vi "paper1.vi"() -> ()   [LabVIEW 2019]
uses:
  <vilib>/BLE/type_def/address_type.ctl
panel:
  out "check time elapsed (S)":dbl
  in  "Tab Control":T1(tab)
  in  "both 3":path=path "C:/Users/Admin/Desktop/Asfand/Working Examples dont edit/7_audio random indicator/both.wav"
  in  "left 2":path=path "C:/Users/Admin/Desktop/Asfand/Working Examples dont edit/7_audio random indicator/left.wav"
  in  "right 3":path=path "C:/Users/Admin/Desktop/Asfand/Working Examples dont edit/7_audio random indicator/right.wav"
  out "BLED112 Dongle Info":string
  in  "COM Bluegiga in":refnum<visa-resource-name>="COM3"
  in  "Address Type":T2=1 items=["Public", "Random"]
  in  "MAC Address":string="F7:AE:10:9A:D9:38"
  out "Scanning":bool
  out "Connected":bool
  out "User input history":string[](array[string])
  out "right 4":i16[](array[numeric])
  out "left 3":i16[](array[numeric])
  out "both":i16[](array[numeric])
  out "Seconds that the game lasted.":dbl
  out "total commands":i32
  out "timer started?":bool
  in  "savefile":path=path "C:/Users/Admin/Desktop/experiment results/name_test1.xlsx" caption="Filename"
  out "possible decisions":string[](array[string])
  out "result":i16
  out "uuid loop":i32
  out "stimulii section precursor":bool
  out "LARGE LOOP":i32
  out "INSIDE RANDOM LOOP":i16
  out "Post trigger response?":bool
  out "Trigger checked?":bool
  out "UUID START":bool
  out "Stimulii section":bool
  out "Stimulii Given?":bool
  out "Number of moves loop":i32
  in  "Right threshold real time update":dbl(slide)=40.2088948787062 scale=0.0..255.0
  out "right":u8(graph)
  out "left":u8(graph)
  out "Left Eye element (PIN A0)":u8
  out "Right Eye Element (PIN A1)":u8
  out "DECISION LOOP":i32
  out "last eye movement":string
  out "Post-Trigger Detection":string
  in  "left threshod real time update":dbl(slide)=40.58355437665783 scale=0.0..255.0
  out "Game finished?":bool=TRUE
  out "Trigger  right eye":bool
  out "right-":bool
  out "Left-":bool
  out "both-":bool
  out "Both":bool
  out "Left":bool
  out "Right":bool
  # "1.Blink both eyes to initiate trigger,\n then blink as stimulii.\n2. If the led user input led does not turn on. \n(try blinking again, a faster response can do the trick)\n3. There will be 20 commands. \n4. moving your head will triger a response.  (slow and small movment will not)\n5. When 20 commands are registered (with triggers) then game finished \nwill turn red"
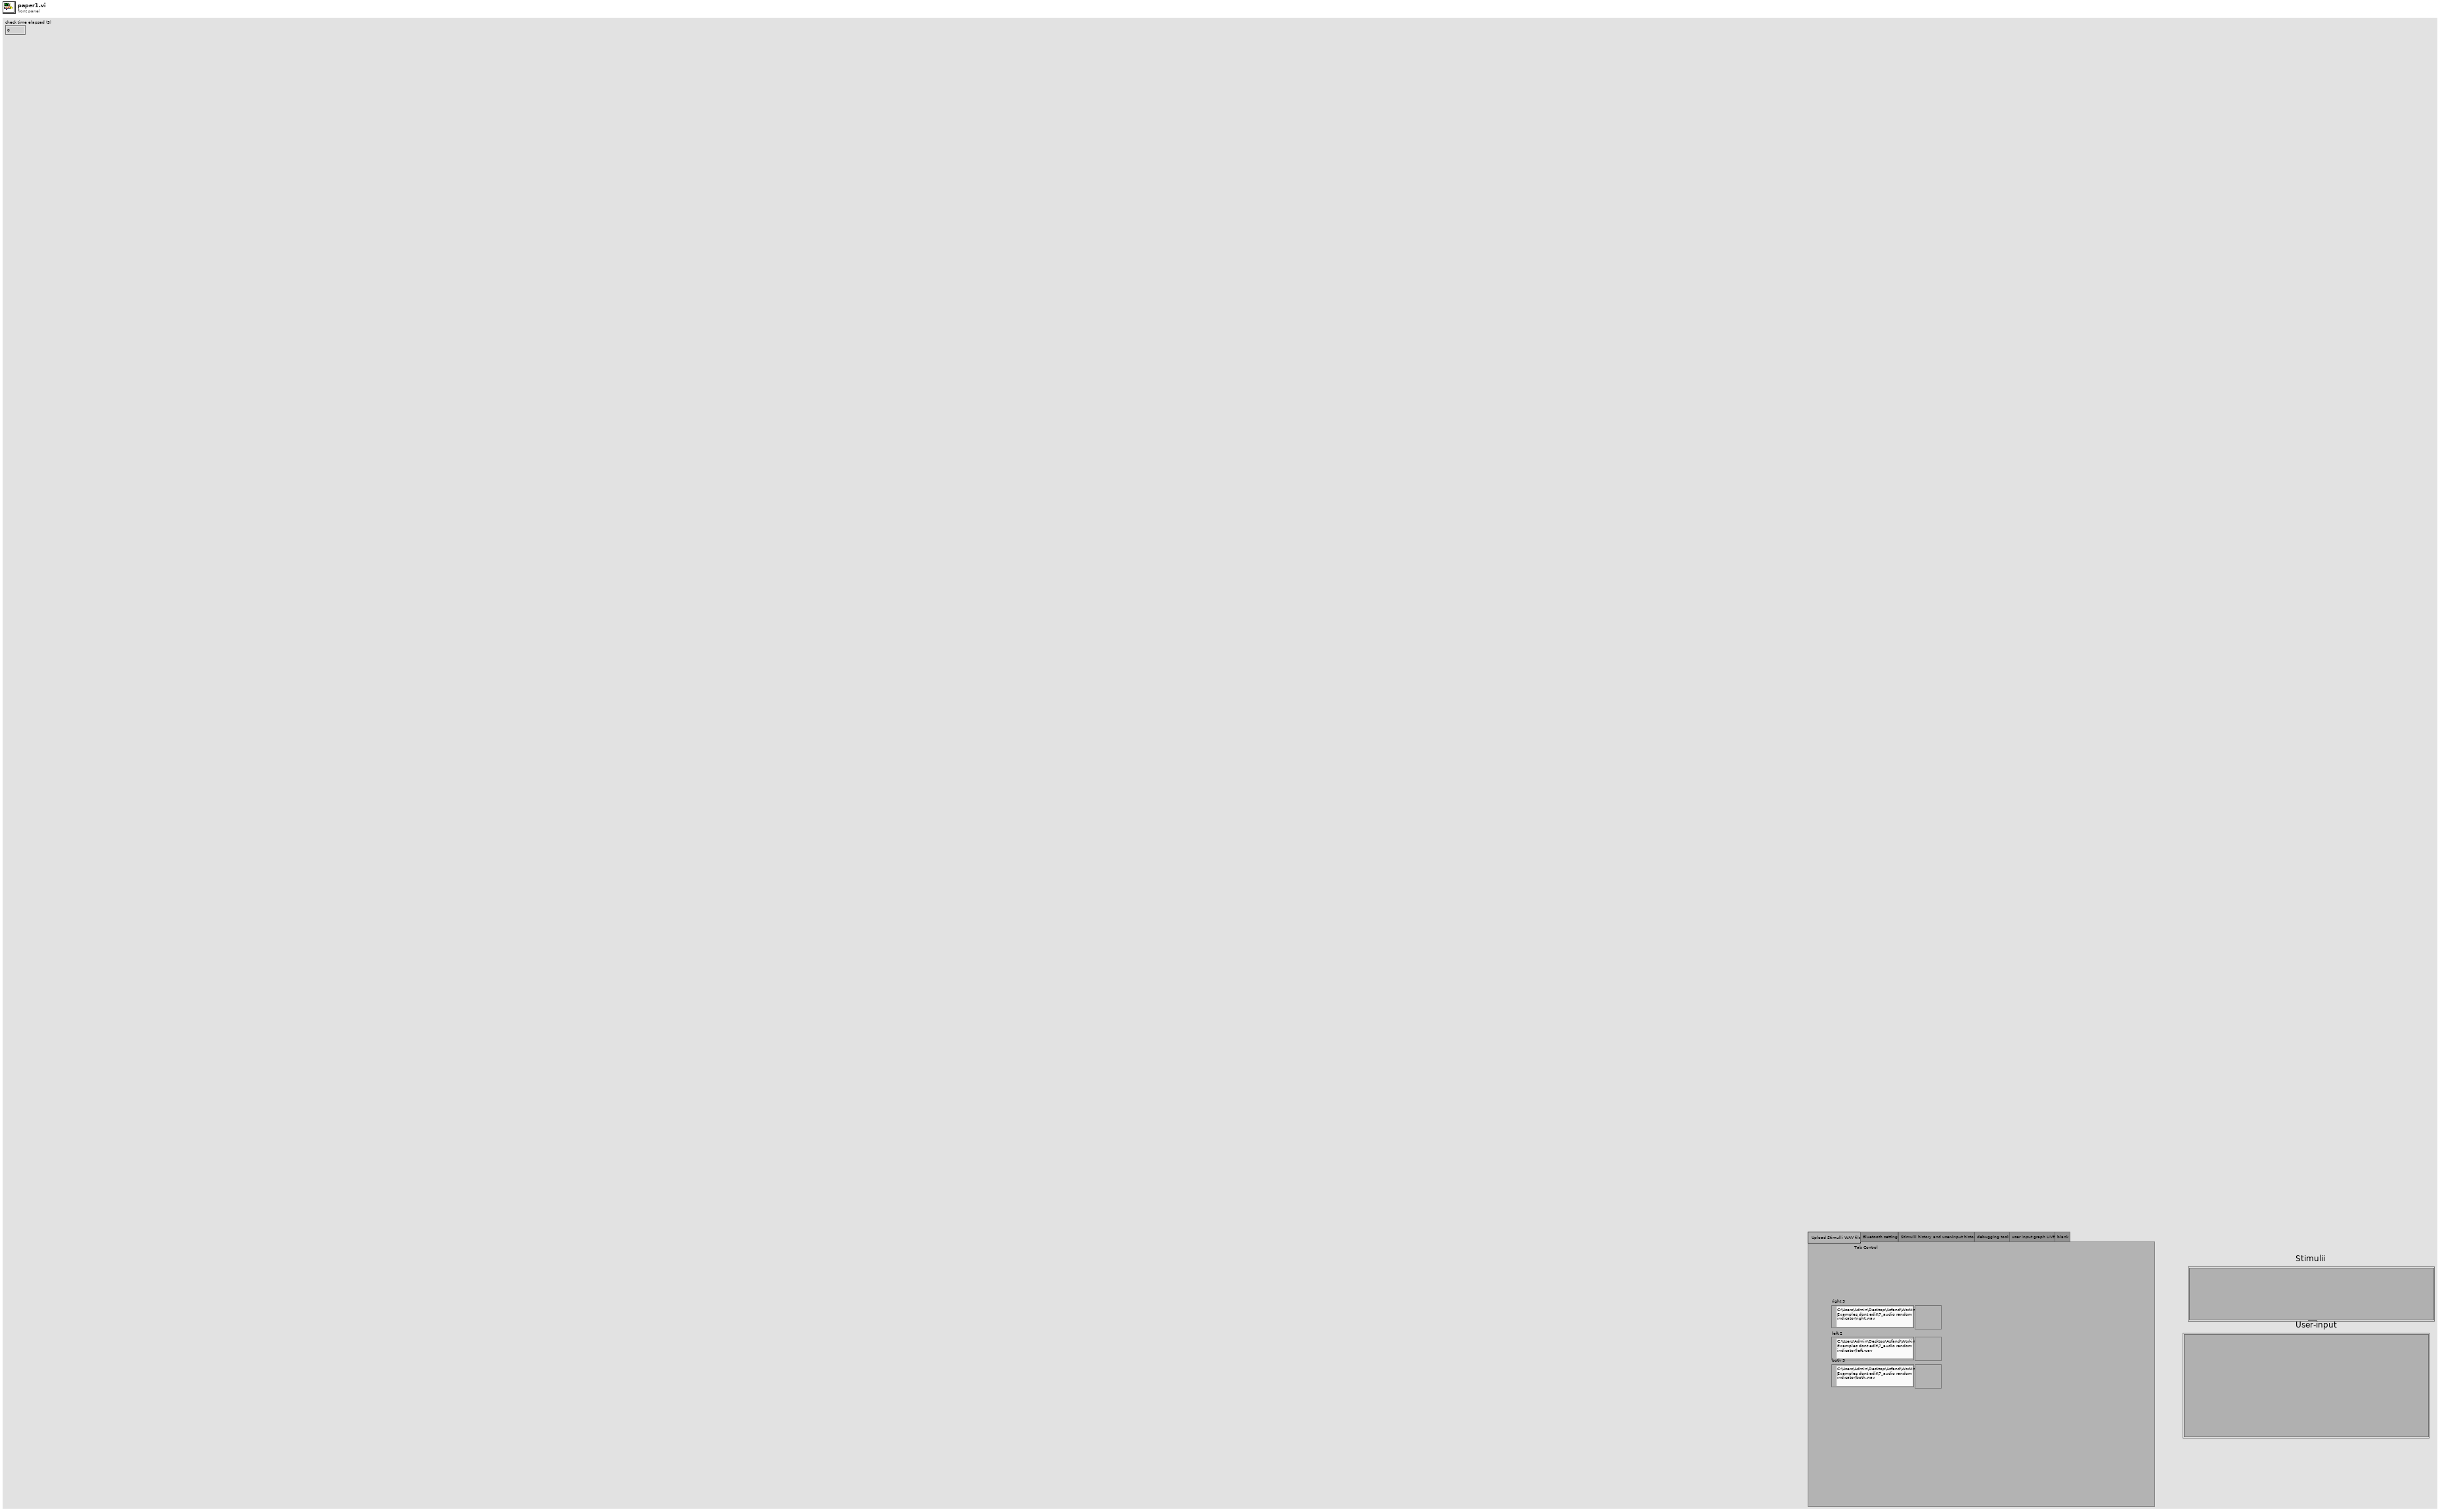
[diagram p1: front panel]
types:
  T1 = enum32{"Upload Stimulli WAV file ", "Bluetooth setting", "Stimulii history and user-input history", "debugging tools", "user input graph LIVE", "blank"}
  T2 = typedef "address_type.ctl" = u8
  T3 = typedef "connection_status_bundle.ctl" = cluster{"MAC Address":string, "cnx handle":u8, "cnx flags":u8, "Address Type":T2, "Connection Interval (ms)":u16, "Timeout(ms)":u16, "Latency":u16, "bonding handle":u8}
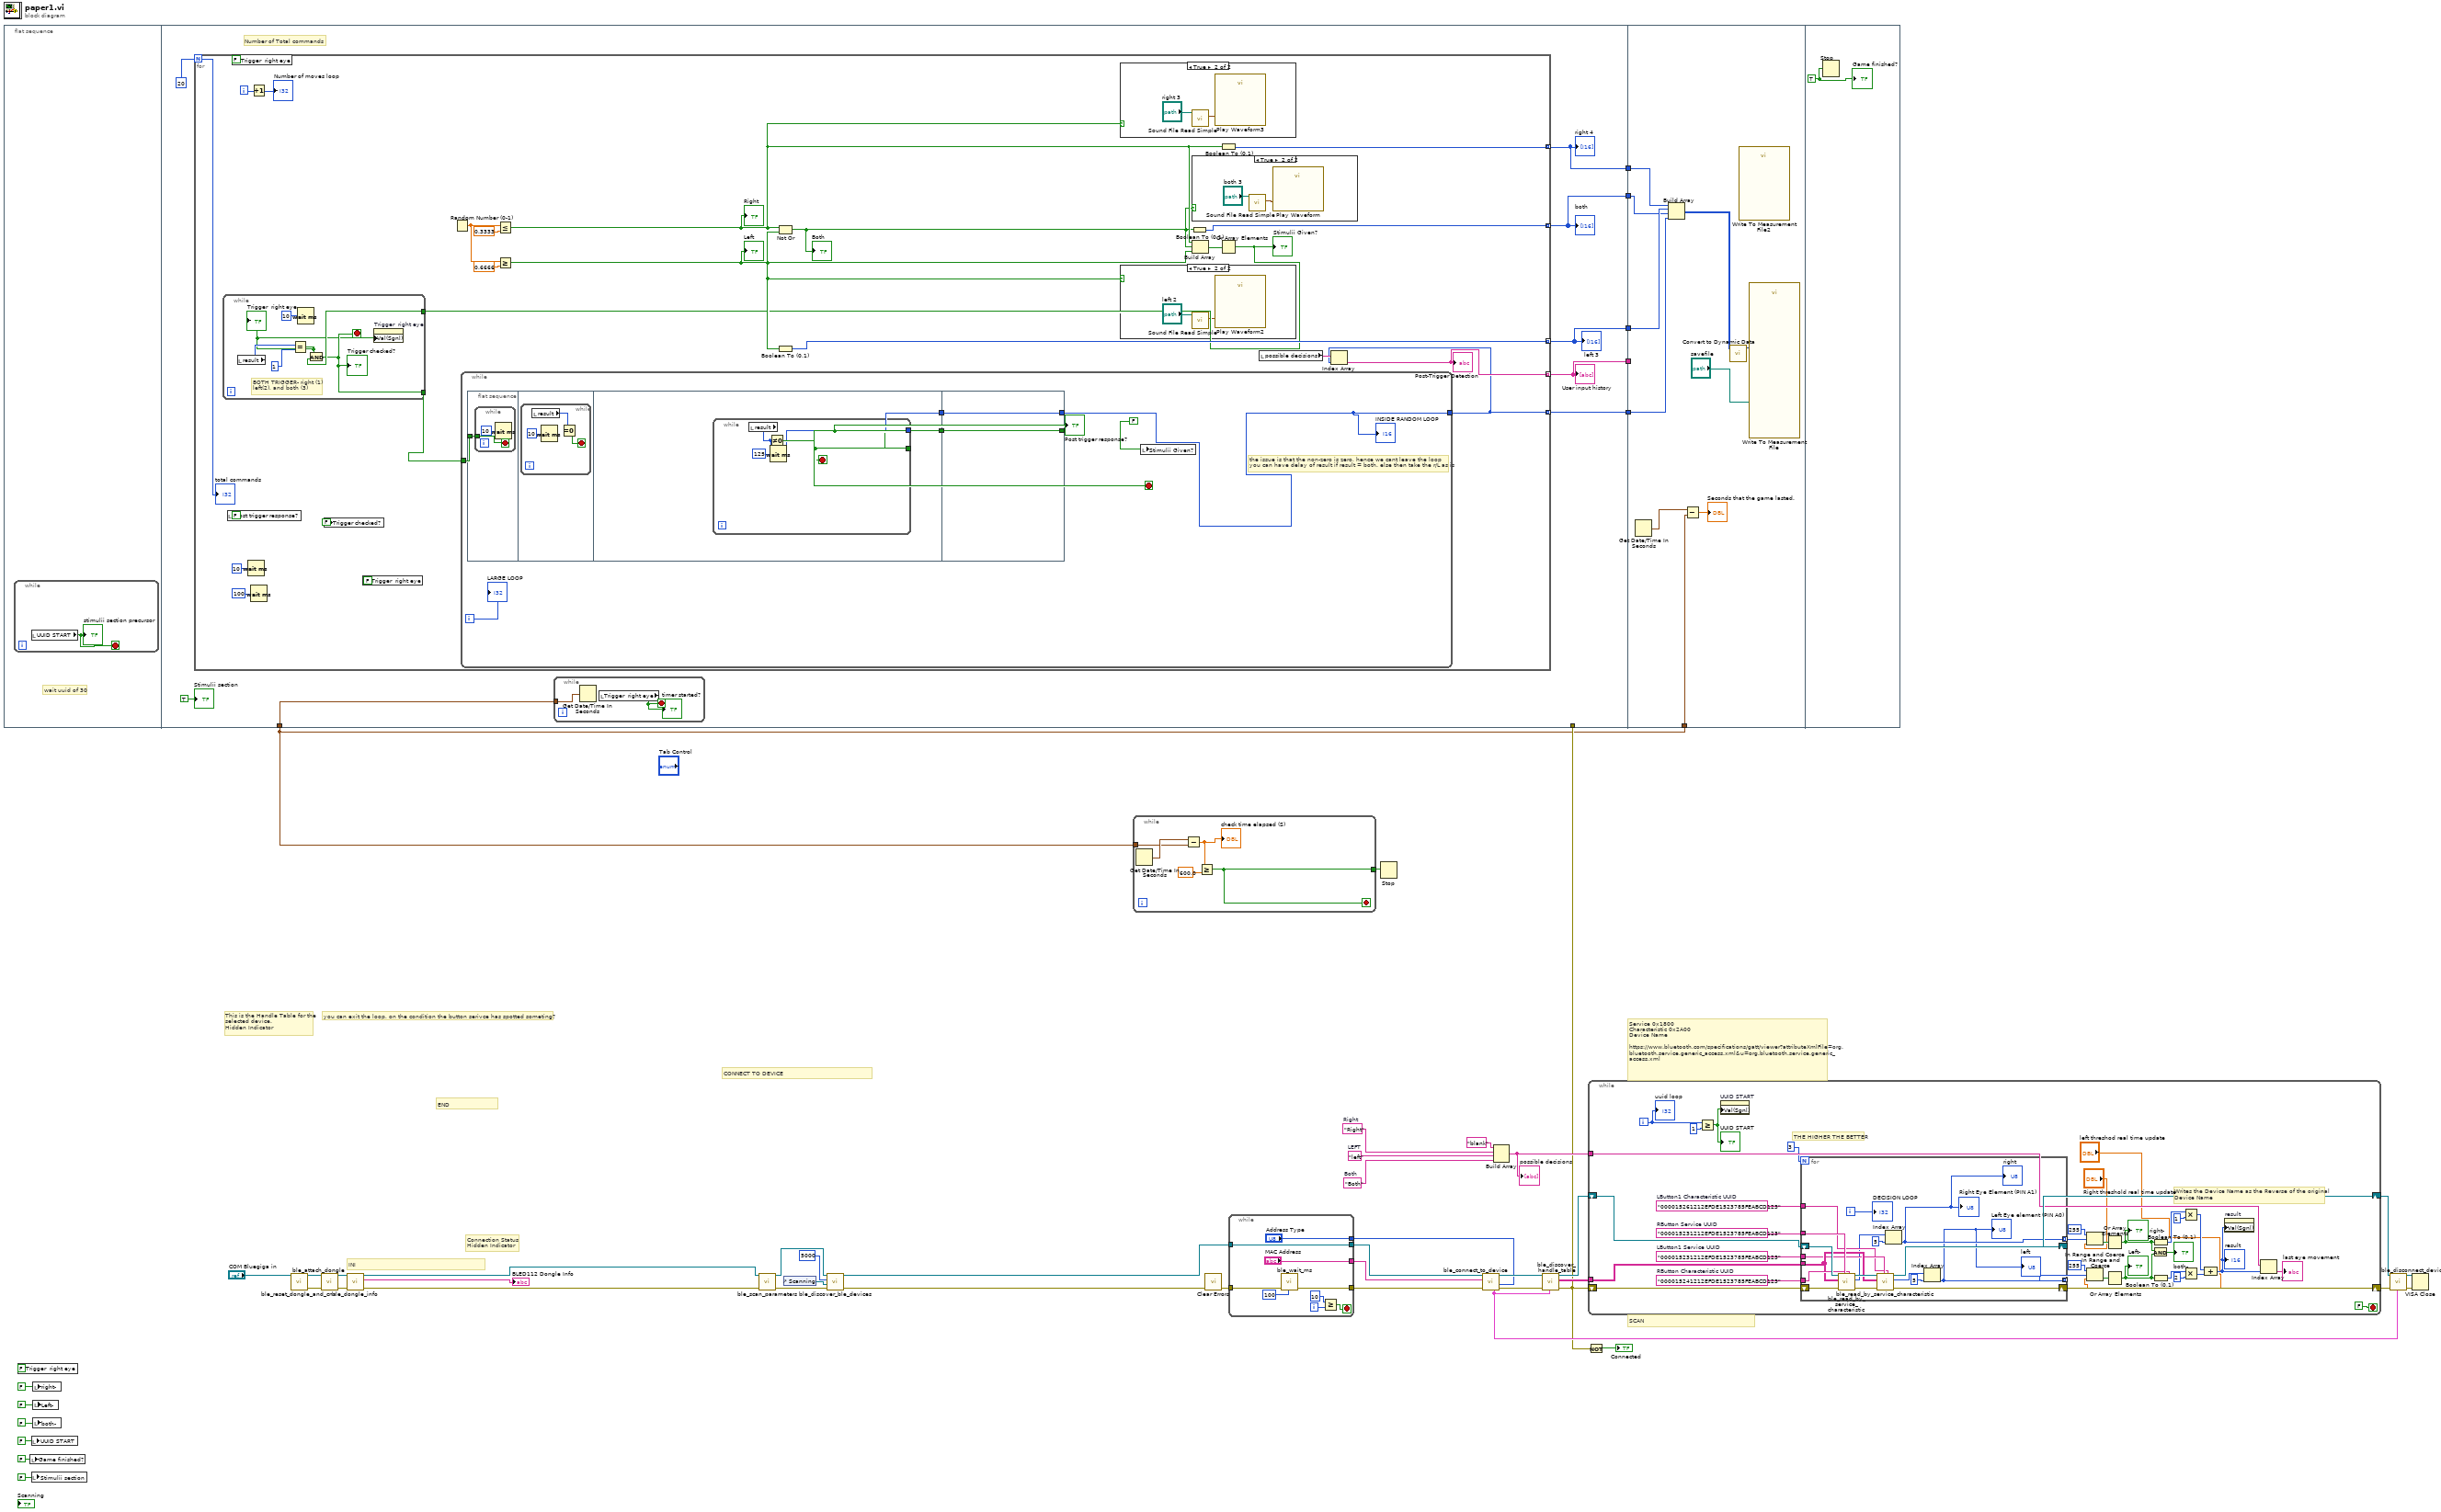
[diagram p0: block diagram]
diagram:
  w16 = "Both"  # Both
  w17 = "left"  # LEFT
  w18 = "Right"  # Right
  # "This is the Handle Table for the\nselected device. \nHidden Indicator"
  # "Service 0x1800\nCharacteristic 0x2A00\nDevice Name\n\nhttps://www.bluetooth.com/specifications/gatt/viewer?attributeXmlFile=org.bluetooth.service.generic_access.xml&u=org.bluetooth.service.generic_access.xml"
  # "CONNECT TO DEVICE"
  # "SCAN"
  # "INI"
  # "you can exit the loop, on the condition the button serivce has spotted someting?"
  # "Connection Status\nHidden Indicator"
  # "END"
  n1 = flat-sequence {
    tunnel: w12 -> [_]
    tunnel: [w56] -> w2
    tunnel: [w55] -> w7
    tunnel: [w54] -> w6
    tunnel: [w53] -> w5
    tunnel: [w52] -> w4
    tunnel: [w51] -> w3
    tunnel: w2 -> [w126]
    tunnel: w7 -> [_]
    tunnel: w6 -> [w123]
    tunnel: w5 -> [w121]
    tunnel: w4 -> [w122]
    tunnel: w3 -> [w120]
    frame #0 {
      # "wait uuid of 30"
      n2 = while {
        stop <- w50 stop-if-true
        n3 = local read "UUID START"() -> (w50:bool)
        "stimulii section precursor" <- w50
      }
    }
    frame #1 {
      # "Number of Total commands"
      n4 = for {
        N: 20 -> [w76]
        tunnel: [w84] -> w54 mode=indexing
        tunnel: [w83] -> w53 mode=indexing
        tunnel: [w80] -> w52 mode=indexing
        tunnel: [w78] -> w55 mode=indexing
        tunnel: [w61] -> w51 mode=indexing
        i -> [w82]
        n5 = local write "Post trigger response?"(FALSE ("non zero")) -> ()
        n6 = local write "Trigger  right eye"(FALSE ("access")) -> ()
        n7 = Wait (ms)(milliseconds to wait=u32 10) -> ()  [unwired: 1 out]
        n8 = Increment(x=w82) -> (x+1=→"Number of moves loop":i32)
        n9 = Wait (ms)(milliseconds to wait=u32 100) -> ()  [unwired: 1 out]
        n10 = local write "Trigger checked?"(FALSE ("end loop")) -> ()
        n11 = local write "Trigger  right eye"(FALSE ("Trigger")) -> ()
        n12 = Random Number (0-1)() -> (number: 0 to 1=w74:dbl)
        n13 = Less Or Equal?(x=w74, y=0.3333) -> (x <= y?=w71:bool)
        "Right" <- w71
        n14 = Greater Or Equal?(x=w74, y=0.6666) -> (x >= y?=w70:bool)
        "Left" <- w70
        n15 = Not Or(1:w70, 2:w71) -> (0:w69:bool)
        "Both" <- w69
        n16 = Boolean To (0,1)(Boolean=w70) -> (0, 1=w80:i16)
        n17 = case shown="True" w71 {
          frame False {
          }
          frame True {
            n18 = call <vilib>:"Sound File Read Simple.vi"("path"="right 3") -> ("data"=w111:waveform(dbl)[])  [unwired: 7 in, 3 out]
            n19 = call "Play Waveform3"("Data"=w111) -> ()  [unwired: 18 in, 1 out]
          }
        }
        n20 = case shown="True" w70 {
          frame False {
          }
          frame True {
            n21 = call <vilib>:"Sound File Read Simple.vi"("path"="left 2") -> ("data"=w113:waveform(dbl)[])  [unwired: 7 in, 3 out]
            n22 = call "Play Waveform2"("Data"=w113) -> ()  [unwired: 18 in, 1 out]
          }
        }
        n23 = Boolean To (0,1)(Boolean=w69) -> (0, 1=w83:i16)
        n24 = case shown="True" w69 {
          frame False {
          }
          frame True {
            n25 = call <vilib>:"Sound File Read Simple.vi"("path"="both 3") -> ("data"=w115:waveform(dbl)[])  [unwired: 7 in, 3 out]
            n26 = call "Play Waveform"("Data"=w115) -> ()  [unwired: 18 in, 1 out]
          }
        }
        n27 = Build Array(w71, w69, w70) -> (w81:bool[])
        n28 = Boolean To (0,1)(Boolean=w71) -> (0, 1=w84:i16)
        n29 = Or Array Elements(Boolean array=w81) -> (logical OR=w65:bool)
        "Stimulii Given?" <- w65
        n30 = while {
          tunnel: [w106] -> w67
          tunnel: w65 -> [w107]
          stop <- w106 stop-if-true
          # "BOTH TRIGGER- right (1)\nleft(2), and both (3)"
          n31 = local read "result"() -> (w110:i16)
          n32 = Equal?(x=w110, y=i16 1) -> (x = y?=w105:bool)
          "Trigger  right eye" <- w105
          n33 = Wait (ms)(milliseconds to wait=u32 10) -> ()  [unwired: 1 out]
          n34 = And(x=w105, y=w107) -> (x .and. y?=w106:bool)
          "Trigger checked?" <- w106
          n35 = property on="Trigger  right eye" class="Bool (strict)"("Val(Sgnl)"=w105) -> ()  [unwired: 2 in, 2 out]
        }
        n36 = while {
          tunnel: w67 -> [w89]
          tunnel: [w85] -> w61
          i -> [w91]
          stop <- w88 stop-if-true
          # "the issue is that the non-zero is zero, hence we cant leave the loop\nyou can have delay of result if result = both. else then take the r/L as is"
          n37 = flat-sequence {
            tunnel: w89 -> [w92]
            tunnel: [w99] -> w87
            tunnel: [w98] -> w86
            tunnel: [w103] -> w85
            tunnel: [w104] -> w88
            tunnel: w87 -> [w104]
            tunnel: w86 -> [w103]
            frame #0 {
              n38 = while {
                tunnel: w92 -> [w94]
                stop <- w94 stop-if-true
                n39 = Wait (ms)(milliseconds to wait=u32 10) -> ()  [unwired: 1 out]
              }
            }
            frame #1 {
              n40 = while {
                stop <- w96 stop-if-true
                n41 = local read "result"() -> (w97:i16)
                n42 = Wait (ms)(milliseconds to wait=u32 10) -> ()  [unwired: 1 out]
                n43 = Equal To 0?(x=w97) -> (x = 0?=w96:bool)
              }
            }
            frame #2 {
              n44 = while {
                tunnel: [w102] -> w99
                tunnel: [w101] -> w98
                stop <- w102 stop-if-true
                n45 = local read "result"() -> (w101:i16)
                n46 = Not Equal To 0?(x=w101) -> (x != 0?=w102:bool)
                n47 = Wait (ms)(milliseconds to wait=u32 125) -> ()  [unwired: 1 out]
              }
            }
            frame #3 {
            }
          }
          n48 = local write "Stimulii Given?"(FALSE ("Stimulii Given?")) -> ()
          "Post trigger response?" <- w88
          "LARGE LOOP" <- w91
          "INSIDE RANDOM LOOP" <- w85
        }
        n49 = local read "possible decisions"() -> (w77:string[])
        n50 = Index Array(array=w77, index=w61) -> (element=w78:string)
        "Post-Trigger Detection" <- w78
        "total commands" <- w76
      }
      "right 4" <- w54
      "left 3" <- w52
      "both" <- w53
      "User input history" <- w55
      n51 = while {
        tunnel: [w60] -> w56
        stop <- w59 stop-if-true
        n52 = Get Date/Time In Seconds() -> (seconds since 1Jan1904=w60:timestamp)
        n53 = local read "Trigger  right eye"() -> (w59:bool)
        "timer started?" <- w59
      }
      "Stimulii section" <- TRUE ("Boolean")
    }
    frame #2 {
      n54 = Get Date/Time In Seconds() -> (seconds since 1Jan1904=w125:timestamp)
      n55 = Build Array(w123, w122, w121, w120) -> (w118:i16[][])
      n56 = Subtract(x=w125, y=w126) -> (x-y=→"Seconds that the game lasted.":dbl)
      n57 = call "Convert to Dynamic Data"("2D Array"=w118) -> ("Dynamic Data Type"=w117:dynamicdata)  [unwired: 3 in]
      n58 = call "Write To Measurement File2"() -> ()  [unwired: 17 in, 3 out]
      n59 = call "Write To Measurement File"("Signals"=w117, "Filename"="savefile") -> ()  [unwired: 15 in, 3 out]
    }
    frame #3 {
      w127 = TRUE
      n60 = Stop(stop? (T)=w127) -> ()
      "Game finished?" <- w127
    }
  }
  n61 = local write "Trigger  right eye"(FALSE ("access")) -> ()
  n62 = local write "Game finished?"(FALSE ("game finished")) -> ()
  n63 = local write "UUID START"(FALSE ("x = y?")) -> ()
  n64 = local write "Stimulii section"(FALSE ("Boolean")) -> ()
  n65 = local write "right-"(FALSE ("right")) -> ()
  n66 = local write "Left-"(FALSE ("Left")) -> ()
  n67 = local write "both-"(FALSE ("both")) -> ()
  n68 = call <vilib>:"ble_reset_dongle_and_cnx.vi"("COM Bluegiga in"="COM Bluegiga in") -> ("error out"=w34:errorcluster, "COM Bluegiga out"=w32:refnum<visa-resource-name>)  [unwired: 9 in]
  n69 = call <vilib>:"ble_attach_dongle.vi"("error in (no error)"=w34, "COM Bluegiga in"=w32) -> ("error out"=w36:errorcluster, "COM Bluegiga out"=w35:refnum<visa-resource-name>)  [unwired: 8 in]
  n70 = call <vilib>:"ble_dongle_info.vi"("error in (no error)"=w36, "COM Bluegiga in"=w35) -> ("error out"=w42:errorcluster, "info"=→"BLED112 Dongle Info":string, "COM Bluegiga out"=w43:refnum<visa-resource-name>)  [unwired: 7 in]
  n71 = call <vilib>:"ble_scan_parameters.vi"("error in (no error)"=w42, "COM Bluegiga in"=w43) -> ("error out"=w40:errorcluster, "COM Bluegiga out"=w41:refnum<visa-resource-name>)  [unwired: 7 in, 1 out]
  n72 = control-ref of="Scanning"() -> (w46:refnum<vi>)
  n73 = call <vilib>:"ble_discover_ble_devices.vi"("error in (no error)"=w40, "LED ref"=w46, "Scan Duration (10000ms)"=u32 5000, "COM Bluegiga in"=w41) -> ("error out"=w30:errorcluster, "COM Bluegiga out"=w47:refnum<visa-resource-name>)  [unwired: 5 in, 1 out]
  n74 = while {
    tunnel: w2 -> [w131]
    tunnel: [w128] -> w1
    stop <- w128 stop-if-true
    n75 = Get Date/Time In Seconds() -> (seconds since 1Jan1904=w132:timestamp)
    n76 = Subtract(x=w132, y=w131) -> (x-y=w130:dbl)
    "check time elapsed (S)" <- w130
    n77 = Greater Or Equal?(x=w130, y=600.0) -> (x >= y?=w128:bool)
  }
  n78 = call <vilib>:"Clear Errors.vi"("error in (no error)"=w30) -> ("error out"=w29:errorcluster)  [unwired: 5 in, 1 out]
  n79 = while {
    tunnel: w29 -> [w141]
    tunnel: [w140] -> w45
    tunnel: w47 -> [w140]
    tunnel: [w139] -> w44
    tunnel: ["MAC Address"] -> w37
    tunnel: ["Address Type"] -> w28
    i -> [w134]
    stop <- w135 stop-if-true
    n80 = call <vilib>:"ble_wait_ms.vi"("milliseconds to wait (100)"=u32 100, "error in (no error)"=w141) -> ("error out"=w139:errorcluster)  [unwired: 9 in]
    n81 = Greater Or Equal?(x=10, y=w134) -> (x >= y?=w135:bool)
  }
  n82 = Stop(stop? (T)=w1) -> ()
  n83 = call <vilib>:"ble_connect_to_device.vi"("Address Type"=w28, "error in (no error)"=w44, "MAC Address"=w37, "COM Bluegiga in"=w45) -> ("error out"=w13:errorcluster, "COM Bluegiga out"=w31:refnum<visa-resource-name>, "Connection Status"=w14:T3)  [unwired: 5 in]
  n84 = Build Array("blank" ("f"), w18, w17, w16) -> (w15:string[])
  "possible decisions" <- w15
  n85 = call <vilib>:"ble_discover_handle_table.vi"("Connection Status"=w14, "error in (no error)"=w13, "COM Bluegiga in"=w31) -> ("error out"=w12:errorcluster, "Handle table"=w23:string[][], "COM Bluegiga out"=w24:refnum<visa-resource-name>)  [unwired: 6 in]
  n86 = Not(x=w12) -> (.not. x?=→"Connected":bool)
  n87 = while {
    tunnel: w23 -> [w171]
    shift-right: [w168] -> w26
    shift-left: w12 -> [w167]
    shift-right: [w172] -> w25
    shift-left: w24 -> [w175]
    tunnel: w15 -> [w163]
    i -> [w166]
    stop <- FALSE ("stop") stop-if-true
    w169 = "000015261212EFDE1523785FEABCD123"  # LButton1 Characteristic UUID
    w170 = "000015231212EFDE1523785FEABCD123"  # LButton1 Service UUID
    w173 = "000015241212EFDE1523785FEABCD123"  # RButton Characteristic UUID
    w174 = "000015231212EFDE1523785FEABCD123"  # RButton Service UUID
    # "THE HIGHER THE BETTER"
    # "Writes the Device Name as the Reverse of the original\nDevice Name"
    n88 = Greater Or Equal?(x=w166, y=1) -> (x >= y?=w164:bool)
    "UUID START" <- w164
    n89 = property on="UUID START" class="Bool (strict)"("Val(Sgnl)"=w164) -> ()  [unwired: 2 in, 2 out]
    n90 = for {
      N: 3 -> [_]
      tunnel: w174 -> [w192]
      tunnel: w173 -> [w191]
      tunnel: w171 -> [w188]
      tunnel: w170 -> [w187]
      tunnel: w169 -> [w186]
      tunnel: [w176] -> w153 mode=indexing
      shift-right: [w189] -> w172
      shift-left: w175 -> [w193]
      shift-right: [w184] -> w168
      shift-left: w167 -> [w183]
      tunnel: [w177] -> w148 mode=indexing
      i -> [w178]
      n91 = call <vilib>:"ble_read_by_service_characteristic.vi"("Characteristic UUID"=w191, "Service UUID"=w192, "error in (no error)"=w183, "Handle table"=w188, "COM Bluegiga in"=w193) -> ("error out"=w185:errorcluster, "characteristic value"=w181:u8[], "COM Bluegiga out"=w190:refnum<visa-resource-name>)  [unwired: 4 in]
      n92 = call <vilib>:"ble_read_by_service_characteristic.vi"("Characteristic UUID"=w186, "Service UUID"=w187, "error in (no error)"=w185, "Handle table"=w188, "COM Bluegiga in"=w190) -> ("error out"=w184:errorcluster, "characteristic value"=w182:u8[], "COM Bluegiga out"=w189:refnum<visa-resource-name>)  [unwired: 4 in]
      n93 = Index Array(array=w181, index=5) -> (element=w177:u8)
      "Right Eye Element (PIN A1)" <- w177
      "right" <- w177
      n94 = Index Array(array=w182, index=5) -> (element=w176:u8)
      "Left Eye element (PIN A0)" <- w176
      "left" <- w176
      "DECISION LOOP" <- w178
    }
    n95 = In Range and Coerce(upper limit=u8 255, x=w148, lower limit="Right threshold real time update") -> (In Range?=w147:bool[])  [unwired: 1 out]
    n96 = In Range and Coerce(upper limit=u8 255, x=w153, lower limit="left threshod real time update") -> (In Range?=w152:bool[])  [unwired: 1 out]
    n97 = Or Array Elements(Boolean array=w147) -> (logical OR=w151:bool)
    "right-" <- w151
    n98 = Or Array Elements(Boolean array=w152) -> (logical OR=w150:bool)
    "Left-" <- w150
    n99 = Boolean To (0,1)(Boolean=w151) -> (0, 1=w157:i16)
    n100 = And(x=w151, y=w150) -> (x .and. y?=→"both-":bool)
    n101 = Boolean To (0,1)(Boolean=w150) -> (0, 1=w158:i16)
    n102 = Multiply(x=w157, y=i16 1) -> (x*y=w159:i16)
    n103 = Multiply(x=w158, y=i16 2) -> (x*y=w160:i16)
    n104 = Compound Arithmetic op=ADD(w159, w160) -> (w161:i16)
    "result" <- w161
    n105 = property on="result" class="DigNum (strict)"("Val(Sgnl)"=w161) -> ()  [unwired: 2 in, 2 out]
    n106 = Index Array(array=w163, index=w161) -> (element=→"last eye movement":string)
    "uuid loop" <- w166
  }
  n107 = call <vilib>:"ble_disconnect_device.vi"("Connection Status"=w14, "error in (no error)"=w26, "COM Bluegiga in"=w25) -> ("error out"=w38:errorcluster, "COM Bluegiga out"=w39:refnum<visa-resource-name>)  [unwired: 7 in]
  n108 = VISA Close(VISA resource name=w39, error in (no error)=w38) -> ()  [unwired: 1 out]
